vi "ForwardKinematics2DOF.vi"(6 "L1":dbl, 9 "L2":dbl, 10 "theta1":dbl, 11 "theta2":dbl) -> (1 "x2":dbl, 2 "y1":dbl, 3 "x1":dbl, 4 "y2":dbl)   [LabVIEW 2024]
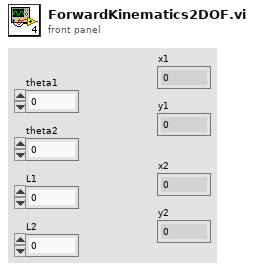
[diagram p1: front panel]
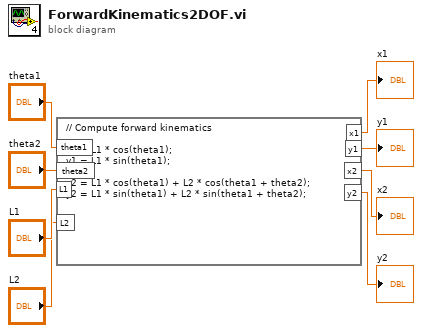
[diagram p0: block diagram]
diagram:
  n1 = formula code="// Compute forward kinematics\n\nx1 = L1 * cos(theta1);\ny1 = L1 * sin(theta1);\n\nx2 = L1 * cos(theta1) + L2 * cos(theta1 + theta2);\ny2 = L1 * sin(theta1) + L2 * sin(theta1 + theta2);"("theta1"="theta1", "theta2"="theta2", "L1"="L1", "L2"="L2") -> ("x1"=→"x1":dbl, "y1"=→"y1":dbl, "x2"=→"x2":dbl, "y2"=→"y2":dbl)
